vi "Draw Horizontal Line.vi"(6 "Colour":u32(colorbox), 9 "Point 2":T1, 10 "Point 1":T1, 11 "Pixels":refnum<data-value>) -> ()   [LabVIEW 2020, in "Raster.lvlib"]
uses:
  Raster.lvlib
  Point 2D.ctl
  <vilib>/Utility/High Resolution Relative Seconds.vi
  Utility/Utility.lvlib
panel:
  out "Processing Time [s]":dbl format="%.1p"
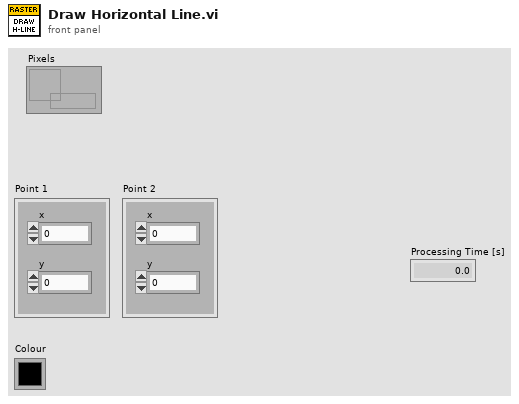
[diagram p1: front panel]
types:
  T1 = typedef "Raster.lvlib/Point 2D.ctl" = cluster{"x":i32, "y":i32}
  T2 = cluster{"pointer":u64, "size_0":u32, "stride_0":i32, "size_1":u32, "stride_1":i32, "element size":u32, "subarray?":bool}
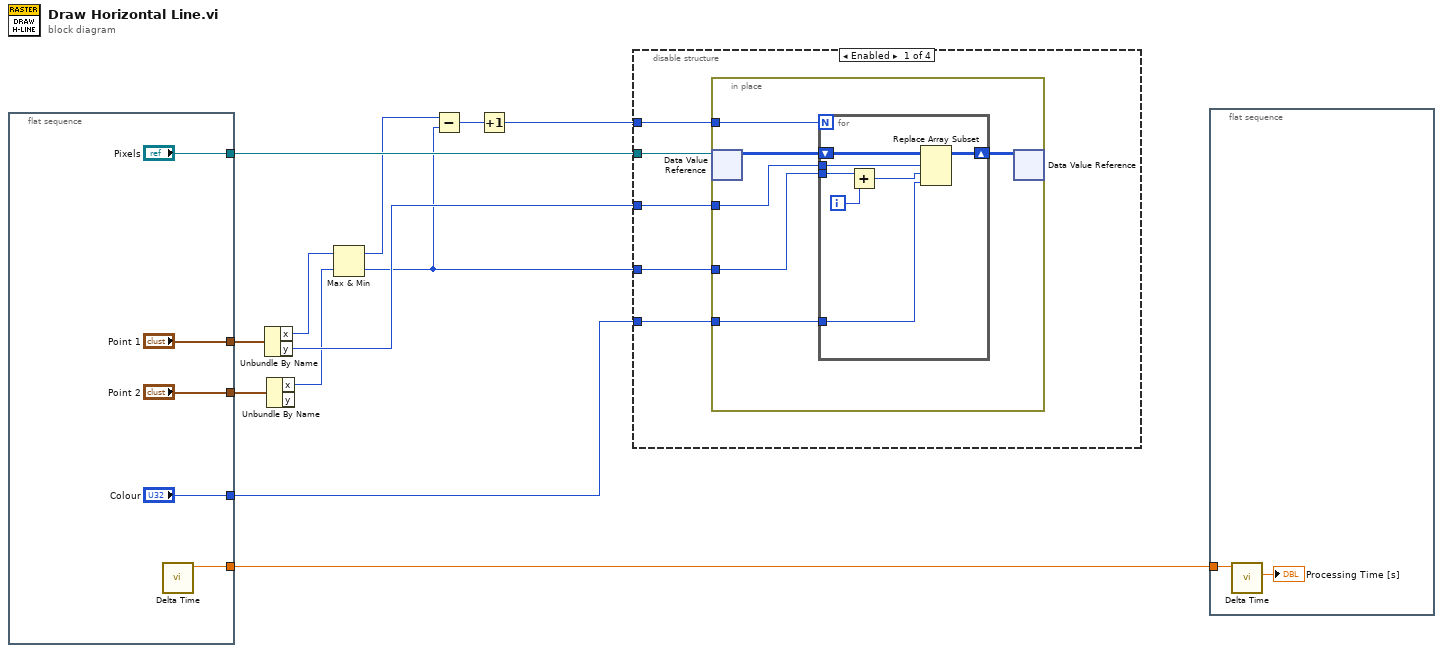
[diagram p0: block diagram]
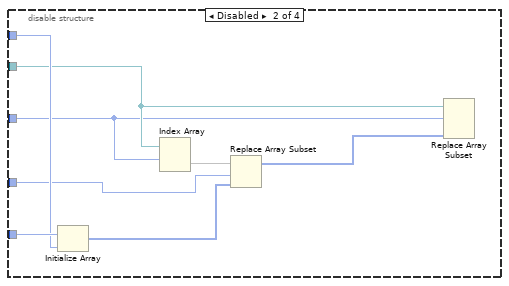
[diagram p2: hidden frame]
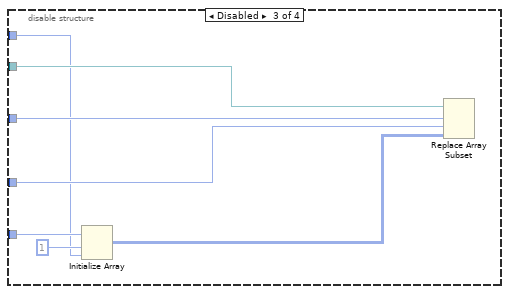
[diagram p3: hidden frame]
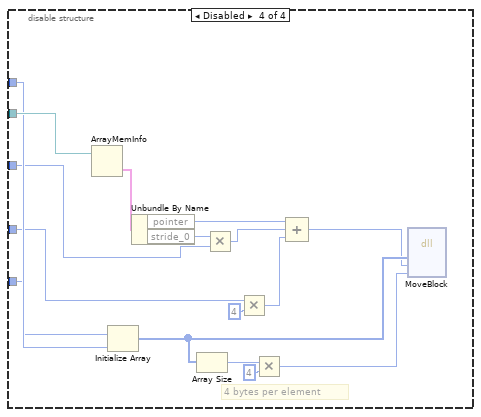
[diagram p4: hidden frame]
diagram:
  n1 = flat-sequence {
    tunnel: ["Point 1"] -> w10
    tunnel: ["Point 2"] -> w9
    tunnel: ["Pixels"] -> w11
    tunnel: ["Colour"] -> w5
    tunnel: [w13] -> w12
    frame #0 {
      n2 = call "Delta Time.vi"() -> ("Relative Seconds Out"=w13:dbl)  [unwired: 10 in, 1 out]
    }
  }
  n3 = Unbundle By Name(w10) -> ("x"=w2:i32, "y"=w7:i32)
  n4 = Unbundle By Name(w9) -> ("x"=w4:i32)  [unwired: 1 out]
  n5 = Max & Min(x=w2, y=w4) -> (max(x,y)=w3:i32, min(x,y)=w1:i32)
  n6 = Subtract(x=w3, y=w1) -> (x-y=w8:i32)
  n7 = Increment(x=w8) -> (x+1=w6:i32)
  n8 = disable-structure shown="Enabled" {
    disable-tunnel: w11 -> [w18 w41 w50 w66]
    disable-tunnel: w7 -> [w22 w37 w49 w58]
    disable-tunnel: w6 -> [w21 w42 w45 w65]
    disable-tunnel: w5 -> [w20 w43 w51 w64]
    disable-tunnel: w1 -> [w19 w38 w48 w55]
    frame Enabled {
      n9 = in-place {
        in-place-border: w22 -> [w28]
        in-place-border: w21 -> [w27]
        in-place-border: w20 -> [w26]
        in-place-border: w19 -> [w25]
        n10 = in-place-dvr #1(w18) -> (w24:u32[][])  [unwired: 1 out]
        n11 = for {
          N: w27 -> [_]
          tunnel: w25 -> [w32]
          tunnel: w28 -> [w30]
          shift-right: [w34] -> w23
          shift-left: w24 -> [w35]
          tunnel: w26 -> [w29]
          i -> [w31]
          n12 = Add(x=w32, y=w31) -> (x+y=w33:i32)
          n13 = Replace Array Subset(array=w35, new element=w29, index (row)=w30, index (col)=w33) -> (w34:u32[][])
        }
        n14 = in-place-dvr #1(w23) -> ()  [unwired: 2 out]
      }
    }
    frame Disabled {
      n15 = Initialize Array(w43, w42) -> (w39:u32[])
      n16 = Index Array(array=w41, index (row)=w37) -> (element=w40)  [unwired: 1 in]
      n17 = Replace Array Subset(array=w40, new element=w39, index=w38) -> (w36:u32[])
      n18 = Replace Array Subset(array=w41, new element=w36, index (row)=w37) -> (w44:u32[])  [unwired: 1 in]
    }
    frame Disabled {
      n19 = Initialize Array(w51, 1 ("dimension size"), w45) -> (w47:u32[][])
      n20 = Replace Array Subset(array=w50, new element=w47, index (row)=w49, index (col)=w48) -> (w52:u32[])
    }
    frame Disabled {
      # "4 bytes per element"
      n21 = ArrayMemInfo(3:w66) -> (0:w68:T2, 1:w67:u32[][])
      n22 = Initialize Array(w64, w65) -> (w63:u32[])
      n23 = Unbundle By Name(w68) -> ("pointer"=w69:u64, "stride_0"=w59:i32)
      n24 = Array Size(array=w63) -> (size(s)=w62:i32)
      n25 = Multiply(x=w59, y=w58) -> (x*y=w57:i32)
      n26 = Multiply(x=w55, y=4) -> (x*y=w54:i32)
      n27 = Multiply(x=w62, y=4) -> (x*y=w60:i32)
      n28 = Compound Arithmetic op=ADD(w69, w57, w54) -> (w53:u64)
      n29 = dll-call lib="LabVIEW" fn="MoveBlock"("Src"=w63, "Dst"=w53, "Size"=w60) -> ()  [unwired: 7 in, 2 out]
    }
  }
  n30 = flat-sequence {
    tunnel: w12 -> [w71]
    frame #0 {
      n31 = call "Delta Time.vi"("Relative Seconds In"=w71) -> ("Delta Time [s]"=→"Processing Time [s]":dbl)  [unwired: 9 in, 1 out]
    }
  }
